vi "Make_Tree_Item.vi"(8 "error in (no error)":errorcluster, 11 "IB_PackedLib in":refnum<class "IB_PackedLib.lvclass">) -> (0 "error out":errorcluster, 3 "TreeSrcItem":refnum<class "IB_Tree_Item_Source.lvclass">)   [LabVIEW 2020, in "IB_PackedLib.lvclass"]
uses:
  <vilib>/AppBuilder/IB_Classes/Source/Container/Build/PackedLib/IB_PackedLib.lvclass
  <vilib>/AppBuilder/IB_Classes/Source/Container/Build/PackedLib/IB_PackedLib.lvclass/IB_PackedLib.ctl
  <vilib>/AppBuilder/IB_Classes/Tree_Item_Source_PackedLib/IB_Tree_Item_Source_PackedLib.lvclass
  e:/builds/penguin/labview/branches/2020/dev/dist/vi.lib/AppBuilder/IB_Classes/Source/Container/Build/IB_Source_Build.lvclass
  e:/builds/penguin/labview/branches/2020/dev/dist/vi.lib/AppBuilder/IB_Classes/Source/Container/IB_Source_Container.lvclass
  e:/builds/penguin/labview/branches/2020/dev/dist/vi.lib/AppBuilder/IB_Classes/Source/IB_Source.lvclass
  e:/builds/penguin/labview/branches/2020/dev/dist/vi.lib/AppBuilder/IB_Classes/Source/Container/Build/PackedLib/IB_PackedLib.lvclass
  e:/builds/penguin/labview/branches/2020/dev/dist/vi.lib/AppBuilder/IB_Classes/Tree_Item_Source_Build/IB_Tree_Item_Source_Build.lvclass
  e:/builds/penguin/labview/branches/2020/dev/dist/vi.lib/AppBuilder/IB_Classes/Tree_Item_Source_Container/IB_Tree_Item_Source_Container.lvclass
  e:/builds/penguin/labview/branches/2020/dev/dist/vi.lib/AppBuilder/IB_Classes/Tree_Item_Source/IB_Tree_Item_Source.lvclass
  e:/builds/penguin/labview/branches/2020/dev/dist/vi.lib/AppBuilder/IB_Classes/Tree_Item/IB_Tree_Item.lvclass
  e:/builds/penguin/labview/branches/2020/dev/dist/vi.lib/AppBuilder/IB_Classes/Tree_Item_Source_PackedLib/IB_Tree_Item_Source_PackedLib.lvclass
  <vilib>/AppBuilder/IB_Classes/Tree_Item_Source/IB_Tree_Item_Source.lvclass
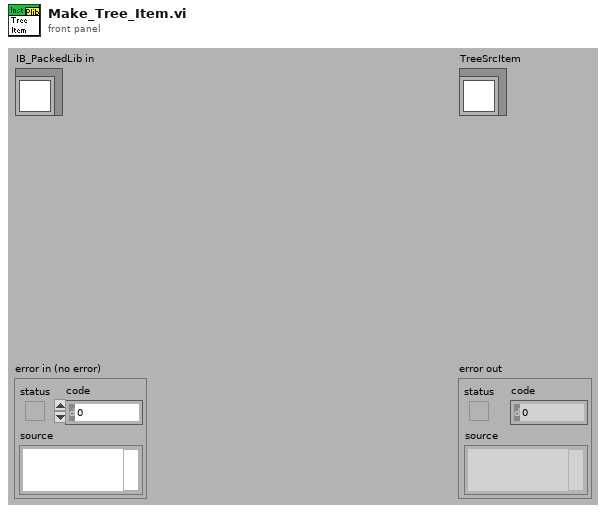
[diagram p1: front panel]
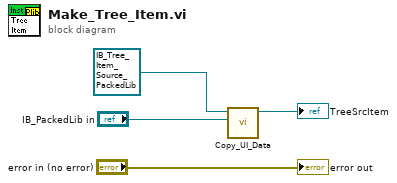
[diagram p0: block diagram]
diagram:
  n1 = call-dynamic "Copy_UI_Data.vi"("IB_Source in"="IB_PackedLib in", "IB_TreeContainerItem.lvclass"=refnum<class "IB_Tree_Item_Source_PackedLib.lvclass"> refnum ("IB_Tree_Item_Source_PackedLib.lvclass")) -> ("IB_TreeContainerItem out"=→"TreeSrcItem":refnum<class "IB_Tree_Item_Source_PackedLib.lvclass">)  [unwired: 1 in, 8 out]
  "error out" <- "error in (no error)"
